vi "subFormDestinationPaths.vi"(0 "Repo Top-Level Path":path, 5 "TestStand Version String":string="[2014, 2016, 2017]", 11 "error in":errorcluster) -> (4 "Repo Top-Level Path out":path, 6 "Program Files Destination Path":path=path "C:/Users/admin/Documents/github/NIVeristandAdd-ons/VeriStand-steps-for-TestStand/Source/Built/ProgramFiles_32/VeriStand Steps for TestStand", 8 "TypePalettes Paths":path[](array[path])=[path "C:/Users/admin/Documents/github/NIVeristandAdd-ons/VeriStand-steps-for-TestStand/Source/Built/documents/National Instruments/TestStand 2014 (32-bit)/Components/TypePalettes", path "C:/Users/admin/Documents/github/NIVeristandAdd-ons/VeriStand-steps-for-TestStand/Source/Built/documents/National Instruments/TestStand 2014 (64-bit)/Components/TypePalettes", path "C:/Users/admin/Documents/github/NIVeristandAdd-ons/VeriStand-steps-for-TestStand/Source/Built/documents/National Instruments/TestStand 2016 (32-bit)/Components/TypePalettes", path "C:/Users/admin/Documents/github/NIVeristandAdd-ons/VeriStand-steps-for-TestStand/Source/Built/documents/National Instruments/TestStand 2016 (64-bit)/Components/TypePalettes", path "C:/Users/admin/Documents/github/NIVeristandAdd-ons/VeriStand-steps-for-TestStand/Source/Built/documents/National Instruments/TestStand 2017 (32-bit)/Components/TypePalettes", path "C:/Users/admin/Documents/github/NIVeristandAdd-ons/VeriStand-steps-for-TestStand/Source/Built/documents/National Instruments/TestStand 2017 (64-bit)/Components/TypePalettes"], 10 "Icon Paths":path[](array[path])=[path "C:/Users/admin/Documents/github/NIVeristandAdd-ons/VeriStand-steps-for-TestStand/Source/Built/documents/National Instruments/TestStand 2014 (32-bit)/Components/Icons", path "C:/Users/admin/Documents/github/NIVeristandAdd-ons/VeriStand-steps-for-TestStand/Source/Built/documents/National Instruments/TestStand 2014 (64-bit)/Components/Icons", path "C:/Users/admin/Documents/github/NIVeristandAdd-ons/VeriStand-steps-for-TestStand/Source/Built/documents/National Instruments/TestStand 2016 (32-bit)/Components/Icons", path "C:/Users/admin/Documents/github/NIVeristandAdd-ons/VeriStand-steps-for-TestStand/Source/Built/documents/National Instruments/TestStand 2016 (64-bit)/Components/Icons", path "C:/Users/admin/Documents/github/NIVeristandAdd-ons/VeriStand-steps-for-TestStand/Source/Built/documents/National Instruments/TestStand 2017 (32-bit)/Components/Icons", path "C:/Users/admin/Documents/github/NIVeristandAdd-ons/VeriStand-steps-for-TestStand/Source/Built/documents/National Instruments/TestStand 2017 (64-bit)/Components/Icons"], 14 "VS Steps Pub Docs Path":path, 15 "error out":errorcluster)   [LabVIEW 2015, in "veristand-steps-build-tools.lvlib"]
uses:
  veristand-steps-build-tools.lvlib
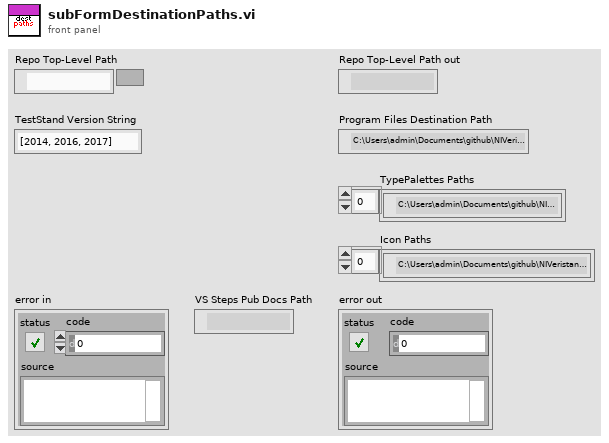
[diagram p1: front panel]
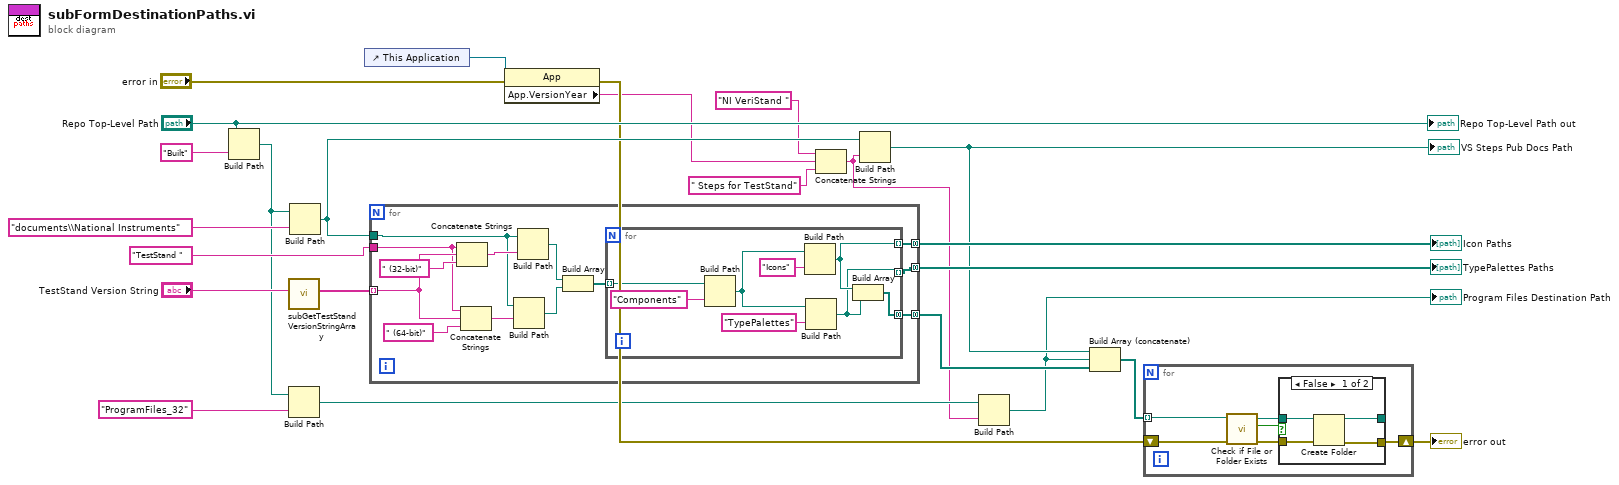
[diagram p0: block diagram]
diagram:
  n1 = Build Path(base path="Repo Top-Level Path", name or relative path="Built") -> (appended path=w16:path)
  n2 = call "subGetTestStandVersionStringArray.vi"("TestStand Version String"="TestStand Version String") -> ("TestStand Version String Array"=w20:string[])  [unwired: 10 in]
  n3 = Build Path(base path=w16, name or relative path="ProgramFiles_32") -> (appended path=w3:path)
  n4 = Build Path(base path=w16, name or relative path="documents\\National Instruments") -> (appended path=w11:path)
  n5 = control-ref of="This Application"() -> (w9:refnum<vi>)
  n6 = for {
    tunnel: w20 -> [w35] mode=indexing
    tunnel: w11 -> [w32]
    tunnel: "TestStand " ("name or relative path") -> [w31]
    tunnel: [w27] -> w14 mode=concatenating
    tunnel: [w26] -> w18 mode=concatenating
    tunnel: [w25] -> w17 mode=concatenating
    n7 = Concatenate Strings(w31, w35, " (32-bit)" ("string")) -> (w33:string)
    n8 = Concatenate Strings(w31, w35, " (64-bit)" ("string")) -> (w34:string)
    n9 = Build Path(base path=w32, name or relative path=w34) -> (appended path=w29:path)
    n10 = Build Path(base path=w32, name or relative path=w33) -> (appended path=w30:path)
    n11 = Build Array(w30, w29) -> (w28:path[])
    n12 = for {
      tunnel: w28 -> [w45] mode=indexing
      tunnel: [w40] -> w27 mode=concatenating
      tunnel: [w39] -> w26 mode=indexing
      tunnel: [w38] -> w25 mode=indexing
      n13 = Build Path(base path=w45, name or relative path="Components") -> (appended path=w42:path)
      n14 = Build Path(base path=w42, name or relative path="Icons") -> (appended path=w39:path)
      n15 = Build Path(base path=w42, name or relative path="TypePalettes") -> (appended path=w38:path)
      n16 = Build Array(w39, w38) -> (w40:path[])
    }
  }
  "Icon Paths" <- w18
  "TypePalettes Paths" <- w17
  n17 = property class="App"(reference=w9, error in="error in") -> (error out=w7:errorcluster, "App.VersionYear"=w5:string)  [unwired: 1 out]
  n18 = Concatenate Strings("NI VeriStand " ("name or relative path"), w5, " Steps for TestStand" ("string")) -> (w2:string)
  n19 = Build Path(base path=w11, name or relative path=w2) -> (appended path=w10:path)
  "VS Steps Pub Docs Path" <- w10
  n20 = Build Path(base path=w3, name or relative path=w2) -> (appended path=w1:path)
  "Program Files Destination Path" <- w1
  n21 = Build Array (concatenate)(w10, w1, w14) -> (w13:path[])
  n22 = for {
    shift-right: [w48] -> w12
    shift-left: w7 -> [w47]
    tunnel: w13 -> [w46] mode=indexing
    n23 = call <vilib>:"Check if File or Folder Exists.vi"("error in (no error)"=w47, "path"=w46) -> ("error out"=w51:errorcluster, "file or folder exists?"=w49:bool, "dup path"=w50:path)  [unwired: 7 in]
    n24 = case shown="False" w49 {
      tunnel: w51 -> [w55 w56]
      tunnel: w50 -> [w54 w57]
      tunnel: [w53 w56] -> w48
      tunnel: [w52 w57] -> _
      frame False {
        n25 = Create Folder(path (use dialog)=w54, error in=w55) -> (created path=w52:path, error out=w53:errorcluster)  [unwired: 1 in, 1 out]
      }
      frame True {
      }
    }
  }
  "error out" <- w12
  "Repo Top-Level Path out" <- "Repo Top-Level Path"
